vi "GetMeasurements.vi"(8 "error in (no error)":errorcluster, 11 "ByteGSAPIBase in":refnum<class "ByteQXAPIBase.lvclass">) -> (0 "error out":errorcluster, 2 "measurements":T1(array[cluster]), 3 "ByteGSAPIBase out":refnum<class "ByteQXAPIBase.lvclass">)   [LabVIEW 2019, in "ByteQXWebAPI.lvlib" / "ByteQXAPIBase.lvclass"]
doc: "Obtain all measurements"
uses:
  ByteQXAPIBase.lvclass
  TypeDef/EditMeasurementReqData.ctl
  Private/module.ctl
  ByteQXAPIBase.lvclass/ByteQXAPIBase.ctl
  <vilib>/Bytelabs/ByteREST/ByteRESTClass/ByteRESTBase/RESTBase.lvclass
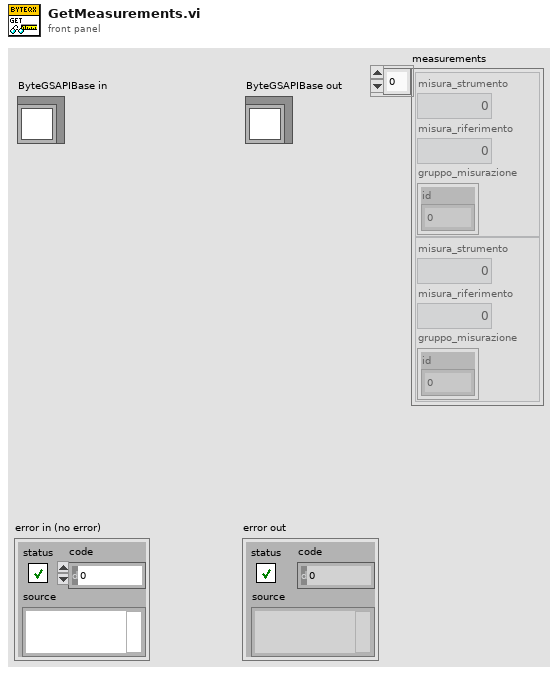
[diagram p1: front panel]
types:
  T1 = cluster{"misura_strumento":sgl, "misura_riferimento":sgl, "gruppo_misurazione":cluster{"id":i32}}[]
  T2 = typedef "ByteQXWebAPI.lvlib/ByteQXAPIBase.lvclass/EditMeasurementReqData.ctl" = cluster{"Id_Group":i32, "misura_strumento":sgl, "misura_riferimento":sgl}
  T3 = typedef "ByteQXWebAPI.lvlib/ByteQXAPIBase.lvclass/module.ctl" = enum16{"gs", "tms"}
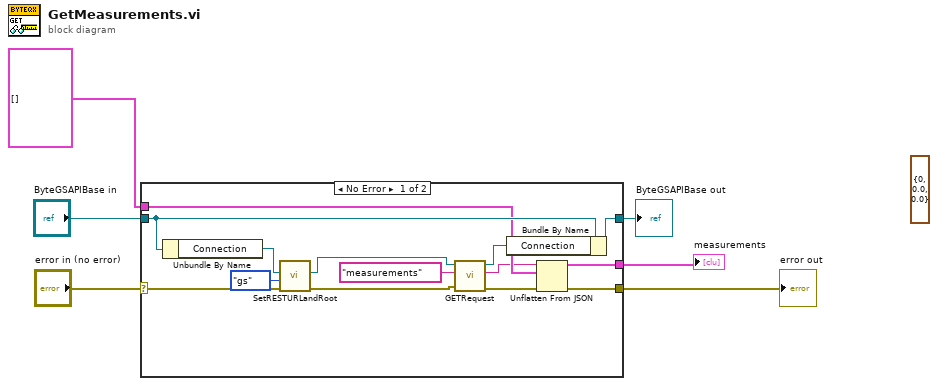
[diagram p0: block diagram]
diagram:
  (unwired) T2 {"Id_Group"=0, "misura_strumento"=0.0, "misura_riferimento"=0.0} ("Valori")
  n1 = case shown="No Error" "error in (no error)" {
    selector: "error in (no error)" -> [w11 w23]
    tunnel: [w15 w23] -> w4
    tunnel: T1 [] ("Valori") -> [w14 w22]
    tunnel: [w13 w22] -> w2
    tunnel: [w18 w21] -> w5
    tunnel: "ByteGSAPIBase in" -> [w20 w21]
    frame No Error {
      n2 = Unbundle By Name(w20) -> ("Connection"=w9:refnum<class "RESTBase.lvclass">)
      n3 = call "SetRESTURLandRoot.vi"("error in (no error)"=w11, "module"=module."gs", "ByteREST in"=w9) -> ("error out"=w10:errorcluster, "ByteREST out"=w8:refnum<class "RESTBase.lvclass">)  [unwired: 7 in]
      n4 = call-dynamic "GETRequest.vi"("error in (no error)"=w10, "Request"="measurements", "ByteRESTBase in"=w8) -> ("error out"=w19:errorcluster, "Body"=w12:string, "ByteRESTBase out"=w17:refnum<class "RESTBase.lvclass">)  [unwired: 5 in, 1 out]
      n5 = Bundle By Name(cluster=w20, "Connection"=w17) -> (w18:refnum<class "ByteQXAPIBase.lvclass">)
      n6 = Unflatten From JSON(JSON string=w12, type and defaults=w14, error in (no error)=w19) -> (value=w13:T1, error out=w15:errorcluster)  [unwired: 4 in]
    }
    frame Error {
    }
  }
  "error out" <- w4
  "ByteGSAPIBase out" <- w5
  "measurements" <- w2
